vi "Windspeed Warnings.vi"() -> ()   [LabVIEW 2012]
doc: "This VI is used to determine the string to output to the weather station based on the current wind and limit settings."
uses:
  Weather Data.ctl
panel:
  out "Weather Data Out":T1={"Current Temperature"=0.0, "Max Temperature"=0.0, "Min Temperature"=0.0, "Temperature Warning?"=FALSE, "Temperature Warning Text"="No Warning", "Current Windspeed"=0.0, "Max Windspeed"=0.0, "Windspeed Warning?"=FALSE, "Windspeed Warning Text"="No Warning"}
  in  "Weather Data In":T1={"Current Temperature"=0.0, "Max Temperature"=0.0, "Min Temperature"=0.0, "Temperature Warning?"=FALSE, "Temperature Warning Text"="No Warning", "Current Windspeed"=0.0, "Max Windspeed"=0.0, "Windspeed Warning?"=FALSE, "Windspeed Warning Text"="No Warning"}
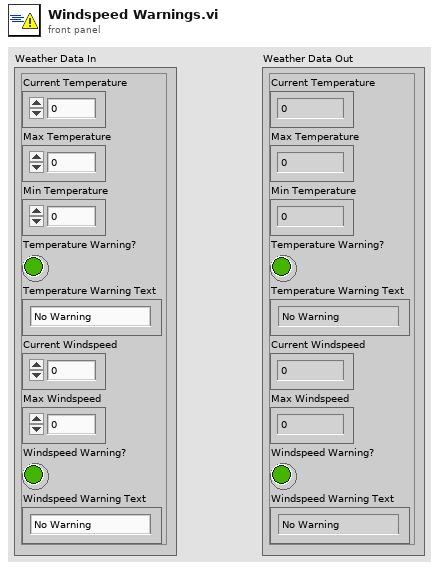
[diagram p1: front panel]
types:
  T1 = typedef "Weather Data.ctl" = cluster{"Current Temperature":dbl, "Max Temperature":dbl, "Min Temperature":dbl, "Temperature Warning?":bool, "Temperature Warning Text":string, "Current Windspeed":dbl, "Max Windspeed":dbl, "Windspeed Warning?":bool, "Windspeed Warning Text":string}
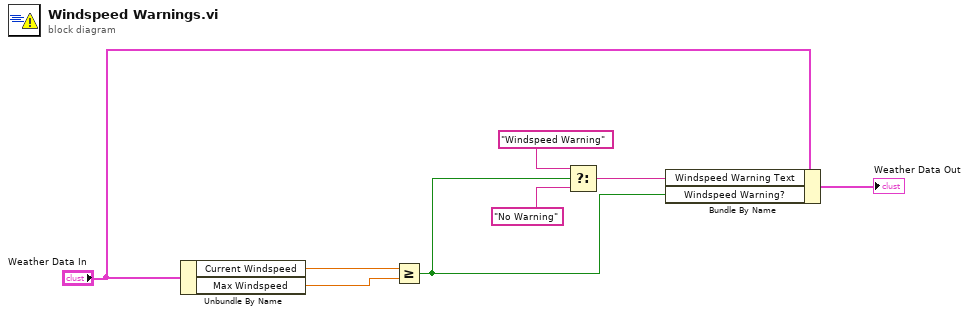
[diagram p0: block diagram]
diagram:
  n1 = Unbundle By Name("Weather Data In") -> ("Current Windspeed"=w8:dbl, "Max Windspeed"=w7:dbl)
  n2 = Greater Or Equal?(x=w8, y=w7) -> (x >= y?=w4:bool)
  n3 = Select(t="Windspeed Warning", s=w4, f="No Warning") -> (s? t:f=w5:string)
  n4 = Bundle By Name(cluster="Weather Data In", "Windspeed Warning Text"=w5, "Windspeed Warning?"=w4) -> (→"Weather Data Out":T1)
